vi "Auto Drive.vi"(1 "Async?":dbl, 3 "Heading":dbl, 4 "Drive Y":dbl, 5 "Turn Power":dbl, 6 "Y Speed":dbl) -> (0 "Done?":bool)   [LabVIEW 2015]
uses:
  Common Code/Drivetrain Commands.ctl
  Common Code/Drivetrain Modes.ctl
  Robot Global Data.vi
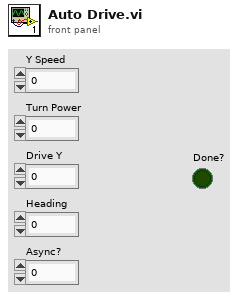
[diagram p1: front panel]
types:
  T1 = typedef "Drivetrain Modes.ctl" = enum16{"Climb", "Manual", "Vision Targeting", "PID Distance Drive", "Hybrid"}
  T2 = typedef "Drivetrain Commands.ctl" = cluster{"Y Power":dbl, "Turn Power":dbl, "1st Gear?":bool, "Modes":T1, "Heading Target":dbl, "X Max Speed":dbl, "Y Max Speed":dbl, "X Min Speed":dbl, "Y Min Speed":dbl, "Y Target":dbl}
  T3 = typedef "Drivetrain Status Cluster.ctl" = cluster{"Modes":T1, "Y (Throttle)":dbl, "X (Steer)":dbl, "Gyro In Range?":bool, "Distance Drive Finished?":bool, "Stop Eject Lockout":bool, "Dist Drive Status":T4, "Y Target":dbl, "Heading Target":dbl, "Vision Target Aligned?":bool, "Gear":dbl, "1st Gear Time":dbl, "2nd Gear Time":dbl, "1st Gear Shifts":dbl, "2nd Gear Shifts":dbl}
  T4 = typedef "Dist Drive Status.ctl" = cluster{"Y In Range":bool, "X In Range":bool, "Gyro In Range":bool, "Y Dist":dbl, "X Dist":dbl, "Gyro":dbl}
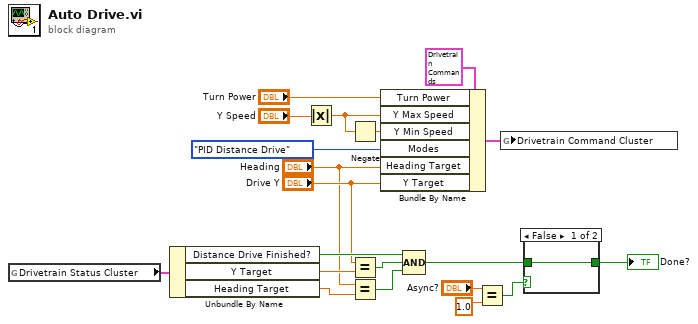
[diagram p0: block diagram]
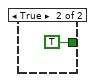
[diagram p2: hidden frame]
diagram:
  n1 = global read "Robot Global Data.vi" "Drivetrain Status Cluster"() -> (w11:T3)
  n2 = Unbundle By Name(w11) -> ("Distance Drive Finished?"=w5:bool, "Y Target"=w4:dbl, "Heading Target"=w3:dbl)
  n3 = Absolute Value(x="Y Speed") -> (abs(x)=w15:dbl)
  n4 = Negate(x=w15) -> (-x=w16:dbl)
  n5 = Equal?(x="Drive Y", y=w4) -> (x = y?=w9:bool)
  n6 = Equal?(x="Heading", y=w3) -> (x = y?=w8:bool)
  n7 = Bundle By Name(cluster=T2 {"Y Power"=0.0, "Turn Power"=0.0, "1st Gear?"=FALSE, "Modes"=enum."Manual", "Heading Target"=0.0, "X Max Speed"=0.0, "Y Max Speed"=0.0, "X Min Speed"=0.0, "Y Min Speed"=0.0, "Y Target"=0.0} ("Drivetrain Command Cluster"), "Turn Power"="Turn Power", "Y Max Speed"=w15, "Y Min Speed"=w16, "Modes"=Drivetrain_Modes."PID Distance Drive", "Heading Target"="Heading", "Y Target"="Drive Y") -> (w19:T2)
  n8 = Compound Arithmetic op=AND(w5, w9, w8) -> (w7:bool)
  n9 = Equal?(x="Async?", y=1.0) -> (x = y?=w13:bool)
  n10 = global write "Robot Global Data.vi" "Drivetrain Command Cluster"(w19) -> ()
  n11 = case shown="False" w13 {
    tunnel: w7 -> [w21 _]
    tunnel: [w21 TRUE] -> w6
    frame False {
    }
    frame True {
    }
  }
  "Done?" <- w6
